vi "Send Terminate.vi"(8 "error in":errorcluster, 11 "ASE Handle":refnum<class "ase.lvclass">) -> (0 "error out":errorcluster, 1 "State":T1, 3 "ASE Handle Duplicate":refnum<class "ase.lvclass">)   [LabVIEW 2024, in "serenial.io-ase.lvlib" / "ase.lvclass"]
doc: "<B>Send the Terminate Signal to the running executable.</B>\n\n<B>This VI will still operate when there is an error at the error-in terminal.</B>\n\nThis VI generates the following errors:\n-5691000: Internal Library Error. Check Error Message for more details.\n1556: Invalid Handle Supplied"
uses:
  ase.lvclass
  Call State.ctl
  ase.lvclass/ase.ctl
  Error Internal Library Implementation Error.vi
  <vilib>/Utility/error.llb/Error Cluster From Error Code.vi
  serenial.io-ase.32.dll
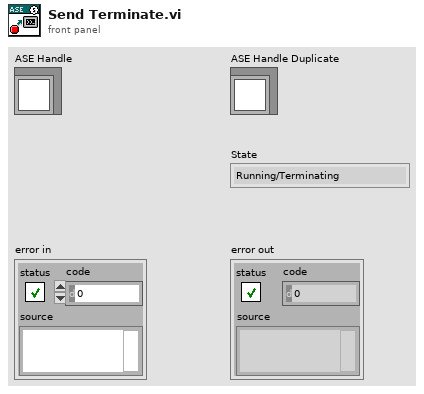
[diagram p1: front panel]
types:
  T1 = typedef "serenial.io-ase.lvlib/ase.lvclass/Call State.ctl" = enum16{"Running/Terminating", "Already Exited"}
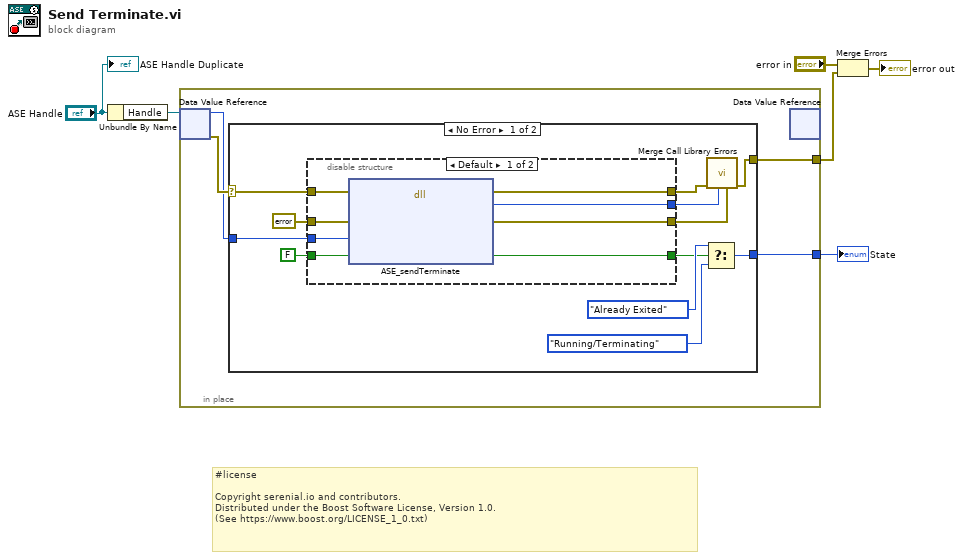
[diagram p0: block diagram]
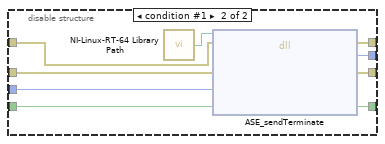
[diagram p2: hidden frame]
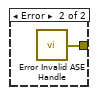
[diagram p3: hidden frame]
diagram:
  # "#license\n\nCopyright serenial.io and contributors.\nDistributed under the Boost Software License, Version 1.0.\n(See https://www.boost.org/LICENSE_1_0.txt)"
  n1 = Unbundle By Name("ASE Handle") -> ("Handle"=w1:refnum<data-value>)
  n2 = in-place "In Place Element Structure" {
    in-place-border: [w9] -> w4
    in-place-border: [w8] -> w3
    n3 = in-place-dvr #1(w1) -> (w7:u64, w10:errorcluster)
    n4 = case shown="No Error" w10 {
      selector: w10 -> [w18 _]
      tunnel: w7 -> [w16 _]
      tunnel: [w22 w40] -> w9
      tunnel: [w19 _] -> w8
      frame No Error {
        n5 = disable-structure shown="Default" {
          disable-tunnel: w18 -> [w30 w38]
          disable-tunnel: errorcluster {"status"=FALSE, "code"=0, "source"=""} ("error") -> [w29 w35]
          disable-tunnel: w16 -> [w28 w34]
          disable-tunnel: FALSE -> [w27 w33]
          disable-tunnel: [w26 w37] -> w14
          disable-tunnel: [w25 w36] -> w13
          disable-tunnel: [w24 w32] -> w12
          disable-tunnel: [w23 w31] -> w11
          frame condition #0 (active) {
            n6 = dll-call lib="C:/Users/marc/code/sift-streaming/labview/Sift/Dependencies/asynchronous-system-exec-v2.0.0/serenial.io-ase/ase/serenial.io-ase.*.*" fn="ASE_sendTerminate"(error in=w30, "Error Out"=w29, "ASE Interface"=w28, "Already Exited"=w27) -> (error out=w26:errorcluster, "Error Code"=w25:i32, "Error Out"=w24:errorcluster, "Already Exited"=w23:bool)  [unwired: 3 in, 1 out]
          }
          frame condition #1 {
            n7 = call "NI-Linux-RT-64 Library Path.vi"() -> ("Path"=w39:path)
            n8 = dll-call lib="?" fn="ASE_sendTerminate"(path in=w39, error in=w38, "Error Out"=w35, "ASE Interface"=w34, "Already Exited"=w33) -> (error out=w37:errorcluster, "Error Code"=w36:i32, "Error Out"=w32:errorcluster, "Already Exited"=w31:bool)  [unwired: 2 in, 1 out]
          }
        }
        n9 = Select(t=Call_State."Already Exited", s=w11, f=Call_State."Running/Terminating" ("State")) -> (s? t:f=w19:T1)
        n10 = call "Merge Call Library Errors.vi"("Library Call Returned Error"=w12, "Error Code"=w13, "error in"=w14) -> ("error IO"=w22:errorcluster)  [unwired: 8 in]
      }
      frame Error {
        n11 = call "Error Invalid ASE Handle.vi"() -> ("Invalid ASE Handle"=w40:errorcluster)
      }
    }
    n12 = in-place-dvr #1() -> ()  [unwired: 1 in, 2 out]
  }
  "State" <- w3
  n13 = Merge Errors("error in", w4) -> (→"error out":errorcluster)
  "ASE Handle Duplicate" <- "ASE Handle"
